vi "Sub_SetNormalCurrent.vi"(0 "Iset":u32, 1 "Channel":i32, 2 "Device Handle":u32) -> ()   [LabVIEW 2013]
uses:
  documentation/SDK/x64_lib/Mightex_LEDDriver_SDK.dll
panel:
  out "Return":i32
  out "Command String":string
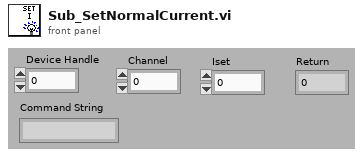
[diagram p1: front panel]
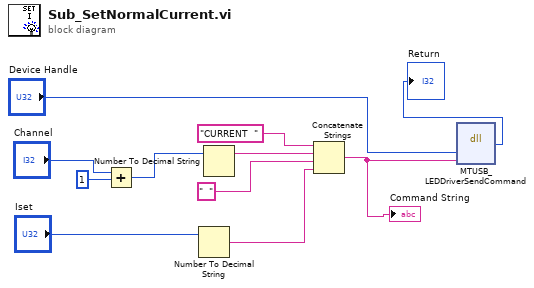
[diagram p0: block diagram]
diagram:
  n1 = Add(x="Channel", y=1) -> (x+y=w3:i32)
  n2 = Number To Decimal String(number="Iset") -> (decimal integer string=w6:string)  [unwired: 1 in]
  n3 = Number To Decimal String(number=w3) -> (decimal integer string=w8:string)  [unwired: 1 in]
  n4 = Concatenate Strings("CURRENT  ", w8, "  ", w6) -> (w2:string)
  "Command String" <- w2
  n5 = dll-call lib="C:/Users/ignacio/Desktop/BIOREACTOR 2/led_control/documentation/SDK/x64_lib/Mightex_LEDDriver_SDK.dll" fn="MTUSB_LEDDriverSendCommand"("arg1"="Device Handle", "arg2"=w2) -> ("return type"=→"Return":i32)  [unwired: 5 in, 2 out]
